vi "Raster Scan_2024-05-21+.vi"() -> ()   [LabVIEW 2024]
doc: "Shows how to move a motor to an absolute position."
uses:
  C:/Users/Behna/OneDrive/Desktop/Kinesis - Move Absolute- my work-with laser - Copy Folder/Thorlabs.MotionControl.Controls.dll
  Thorlabs.MotionControl.Controls.dll
  <vilib>/httpClient/POSTBuffer.vi
  C:/Users/Behna/OneDrive/Desktop/Kinesis - Move Absolute- my work-with laser - Copy Folder/ThorLabs.MotionControl.KCube.DCServoCLI.dll
  ThorLabs.MotionControl.KCube.DCServoCLI.dll
  <vilib>/httpClient/LabVIEWHTTPClient.lvlib
panel:
  out "x*y":dbl
  out "GetMoveAbsolutePositionZ":dbl=6.0
  out "Numeric 2":i32
  out "Numeric":i32
  out "GetMoveAbsolutePositionX":dbl=6.0
  out "x = y?":bool
  in  "initial value_X":dbl=1.0
  in  "initial value_Z":dbl=1.0
  in  "Pulse number":string="5"
  out "body":string="{\"message\":\"success\"}"
  out "headers":string="HTTP/1.1 200 OK\r\nTransfer-Encoding: chunked\r\n\r\n"
  in  "Z-Step size":dbl=1.0
  in  "# Z-points":i32=6
  out "Z-Step":dbl[](array[numeric])=[1.0, 2.0, 3.0, 4.0, 5.0, 6.0]
  out "X-Step":dbl[](array[numeric])=[1.0, 2.0, 3.0, 4.0, 5.0, 6.0]
  in  "# X-points":i32=6
  in  "X-Step size":dbl=1.0
  in  "KCubeDCServoControl 2":refnum<k24>(container)
  in  "SerialNumber 2":string="27261828"
  in  "SerialNumber":string="27261646"
  in  "KCubeDCServoControl":refnum<k24>(container)
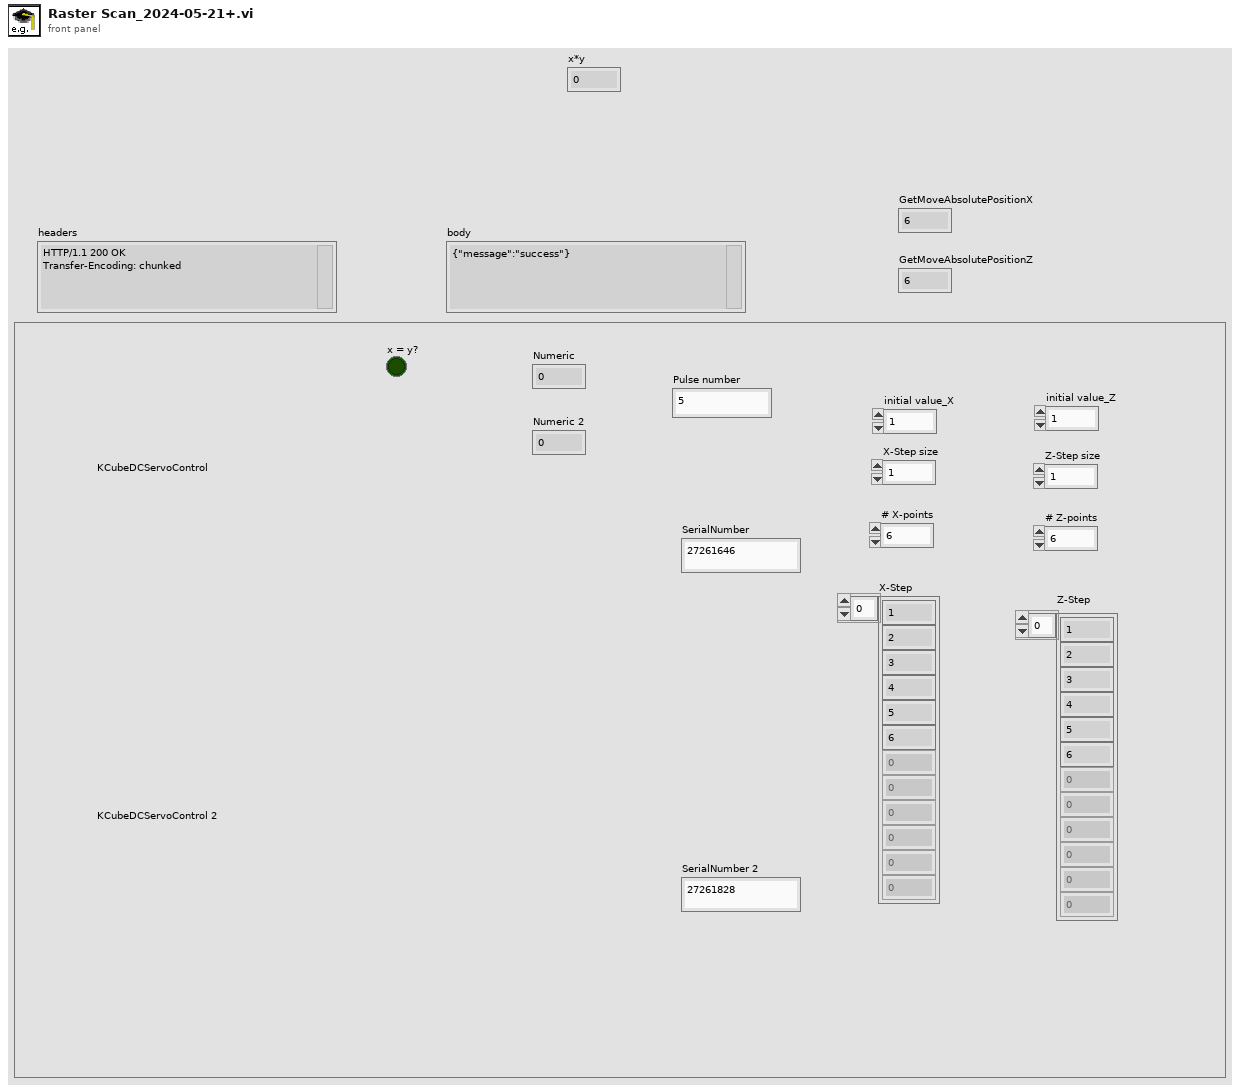
[diagram p1: front panel]
types:
  T1 = typedef "LabVIEWHTTPClient.lvlib/ClientHandle.ctl" = refnum<k1>
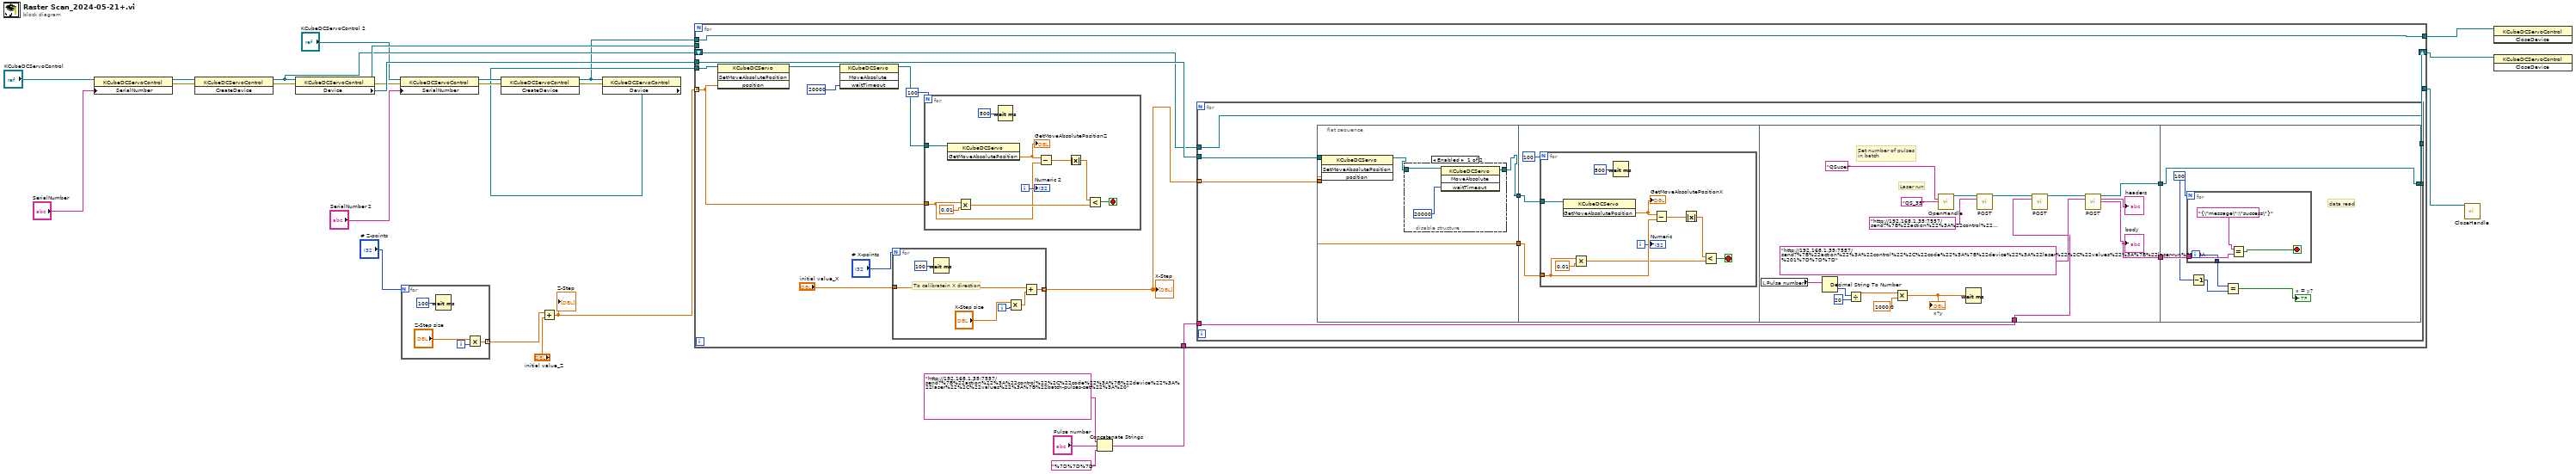
[diagram p0: block diagram]
diagram:
  n1 = property class="KCubeDCServoControl"(reference="KCubeDCServoControl", "SerialNumber"="SerialNumber") -> (reference out=w26:refnum<k24>, error out=w25:errorcluster)  [unwired: 1 in]
  n2 = invoke class="KCubeDCServoControl" method="CreateDevice"(reference=w26, error in=w25) -> (reference out=w20:refnum<k24>, error out=w24:errorcluster)  [unwired: 1 in, 1 out]
  n3 = property class="KCubeDCServoControl"(reference=w20, error in=w24) -> (reference out=w22:refnum<k24>, error out=w12:errorcluster, "Device"=w21:refnum<k24>)
  n4 = property class="KCubeDCServoControl"(reference="KCubeDCServoControl 2", error in=w12, "SerialNumber"="SerialNumber 2") -> (reference out=w15:refnum<k24>, error out=w16:errorcluster)
  n5 = for {
    N: "# Z-points" -> [_]
    tunnel: [w29] -> w3 mode=indexing
    i -> [w30]
    n6 = Wait (ms)(milliseconds to wait=u32 100) -> ()  [unwired: 1 out]
    n7 = Multiply(x="Z-Step size", y=w30) -> (x*y=w29:dbl)
  }
  n8 = invoke class="KCubeDCServoControl" method="CreateDevice"(reference=w15, error in=w16) -> (reference out=w11:refnum<k24>, error out=w17:errorcluster)  [unwired: 1 in, 1 out]
  n9 = Add(x=w3, y="initial value_Z") -> (x+y=w1:dbl[])
  "Z-Step" <- w1
  n10 = property class="KCubeDCServoControl"(reference=w11, error in=w17) -> ("Device"=w13:refnum<k24>)  [unwired: 2 out]
  n11 = Concatenate Strings("http://192.168.1.35:7557/send?%7B%22action%22%3A%22control%22%2C%22code%22%3A%7B%22device%22%3A%22laser%22%2C%22values%22%3A%7B%22batch-pulses-set%22%3A%20" ("string"), "Pulse number", "%7D%7D%7D" ("string")) -> (w4:string)
  n12 = for {
    tunnel: w22 -> [_]
    tunnel: w21 -> [w46]
    shift-right: [w44] -> w19
    shift-left: w20 -> [w45]
    tunnel: w1 -> [w33] mode=indexing
    tunnel: w13 -> [w41]
    tunnel: w11 -> [w40]
    tunnel: [w40] -> w10
    tunnel: [w38] -> w8
    tunnel: w4 -> [w36]
    n13 = invoke class="KCubeDCServo" method="SetMoveAbsolutePosition"(reference=w41, "position"=w33) -> (reference out=w43:refnum<k24>)  [unwired: 2 in, 3 out]
    n14 = invoke class="KCubeDCServo" method="MoveAbsolute"(reference=w43, "waitTimeout"=20000) -> (reference out=w34:refnum<k24>)  [unwired: 2 in, 3 out]
    n15 = for {
      N: "# X-points" -> [_]
      tunnel: [w58] -> w37 mode=indexing
      tunnel: "initial value_X" -> [w57]
      i -> [w61]
      # "To calibratein X direction"
      n16 = Wait (ms)(milliseconds to wait=u32 100) -> ()  [unwired: 1 out]
      n17 = Multiply(x="X-Step size", y=w61) -> (x*y=w59:dbl)
      n18 = Add(x=w57, y=w59) -> (x+y=w58:dbl)
    }
    "X-Step" <- w37
    n19 = for {
      N: 100 -> [_]
      tunnel: w34 -> [w55]
      tunnel: w33 -> [w47]
      i -> [w48]
      stop <- w49 stop-if-true
      n20 = invoke class="KCubeDCServo" method="GetMoveAbsolutePosition"(reference=w55) -> ("GetMoveAbsolutePosition"=w54:dbl)  [unwired: 2 in, 2 out]
      "GetMoveAbsolutePositionZ" <- w54
      n21 = Multiply(x=w47, y=0.01) -> (x*y=w50:dbl)
      n22 = Wait (ms)(milliseconds to wait=u32 500) -> ()  [unwired: 1 out]
      n23 = Subtract(x=w54, y=w47) -> (x-y=w53:dbl)
      n24 = Absolute Value(x=w53) -> (abs(x)=w51:dbl)
      n25 = Less?(x=w51, y=w50) -> (x < y?=w49:bool)
      "Numeric 2" <- w48
    }
    n26 = for {
      tunnel: w46 -> [w71]
      tunnel: w45 -> [w70]
      tunnel: [w70] -> w44
      tunnel: w37 -> [w69] mode=indexing
      tunnel: [w68] -> w38
      tunnel: w36 -> [w66]
      n27 = flat-sequence {
        tunnel: w71 -> [w75]
        tunnel: w69 -> [w72]
        tunnel: [w73] -> w64
        tunnel: [w72] -> w63
        tunnel: w64 -> [w81]
        tunnel: w63 -> [w80]
        tunnel: [w101] -> w67
        tunnel: w66 -> [w99]
        tunnel: [w98] -> w65
        tunnel: [w114] -> w68
        tunnel: w67 -> [w114]
        tunnel: w65 -> [w113]
        frame #0 {
          n28 = invoke class="KCubeDCServo" method="SetMoveAbsolutePosition"(reference=w75, "position"=w72) -> (reference out=w74:refnum<k24>)  [unwired: 2 in, 3 out]
          n29 = disable-structure shown="Enabled" {
            disable-tunnel: w74 -> [w77 _]
            disable-tunnel: [w76 _] -> w73
            frame Enabled {
              n30 = invoke class="KCubeDCServo" method="MoveAbsolute"(reference=w77, "waitTimeout"=20000) -> (reference out=w76:refnum<k24>)  [unwired: 2 in, 3 out]
            }
            frame Disabled {
            }
          }
        }
        frame #1 {
          n31 = for {
            N: 100 -> [_]
            tunnel: w81 -> [w90]
            tunnel: w80 -> [w87]
            i -> [w82]
            stop <- w83 stop-if-true
            n32 = invoke class="KCubeDCServo" method="GetMoveAbsolutePosition"(reference=w90) -> ("GetMoveAbsolutePosition"=w89:dbl)  [unwired: 2 in, 2 out]
            "GetMoveAbsolutePositionX" <- w89
            n33 = Multiply(x=w87, y=0.01) -> (x*y=w84:dbl)
            n34 = Wait (ms)(milliseconds to wait=u32 500) -> ()  [unwired: 1 out]
            n35 = Subtract(x=w89, y=w87) -> (x-y=w88:dbl)
            n36 = Absolute Value(x=w88) -> (abs(x)=w85:dbl)
            n37 = Less?(x=w85, y=w84) -> (x < y?=w83:bool)
            "Numeric" <- w82
          }
        }
        frame #2 {
          # "Set number of pulses \nin batch"
          # "Laser run"
          n38 = local read "Pulse number"() -> (w96:string)
          n39 = Decimal String To Number(string=w96) -> (number=w94:i32)  [unwired: 2 in, 1 out]
          n40 = Divide(x=w94, y=20) -> (x/y=w92:dbl)
          n41 = Multiply(x=w92, y=1000.0) -> (x*y=w95:dbl)
          "x*y" <- w95
          n42 = call <vilib>:"OpenHandle.vi"("username"="QSuser", "password"="QS_35") -> ("client handle out"=w106:T1)  [unwired: 12 in, 1 out]
          n43 = Wait (ms)(milliseconds to wait=w95) -> ()  [unwired: 1 out]
          n44 = call-poly <vilib>:"POST.vi"("client handle"=w106, "url"="http://192.168.1.35:7557/send?%7B%22action%22%3A%22control%22%2C%22code%22%3A%7B%22device%22%3A%22laser%22%2C%22values%22%3A%7B%22batch-mode%22%3A %201%7D%7D%7D") -> ("client handle out"=w105:T1)  [unwired: 10 in, 3 out]
          n45 = call-poly <vilib>:"POST.vi"("client handle"=w105, "url"=w99) -> ("client handle out"=w103:T1)  [unwired: 10 in, 3 out]
          n46 = call-poly <vilib>:"POST.vi"("client handle"=w103, "url"="http://192.168.1.35:7557/send?%7B%22action%22%3A%22control%22%2C%22code%22%3A%7B%22device%22%3A%22laser%22%2C%22values%22%3A%7B%22laser-run%22%3A%201%7D%7D%7D") -> ("client handle out"=w101:T1, "headers"=→"headers":string, "body"=w98:string)  [unwired: 10 in, 1 out]
          "body" <- w98
        }
        frame #3 {
          w110 = 100
          # "data read"
          n47 = for {
            N: w110 -> [_]
            tunnel: w113 -> [w117]
            tunnel: [w115] -> w112
            i -> [w115]
            stop <- w116 stop-if-true
            n48 = Equal?(x="{\"message\":\"success\"}", y=w117) -> (x = y?=w116:bool)
          }
          n49 = Decrement(x=w110) -> (x-1=w111:i32)
          n50 = Equal?(x=w112, y=w111) -> (x = y?=→"x = y?":bool)
        }
      }
    }
  }
  n51 = call <vilib>:"CloseHandle.vi"("client handle"=w8) -> ()  [unwired: 14 in, 1 out]
  n52 = invoke class="KCubeDCServoControl" method="CloseDevice"(reference=w10) -> ()  [unwired: 2 in, 3 out]
  n53 = invoke class="KCubeDCServoControl" method="CloseDevice"(reference=w19) -> ()  [unwired: 2 in, 3 out]
